vi "CrawlingPrechargeState.vi"(8 "error in (no error)":errorcluster, 9 "Cluster in":T2, 10 "Enum in":T1, 11 "Actual Start [i]":i64) -> (0 "error out":errorcluster, 2 "Cluster out":T2, 3 "Enum":T1)   [LabVIEW 2018]
uses:
  Type_Def/Type_Def Actuator Controls.ctl
  Type_Def/Type_Def ControlState.ctl
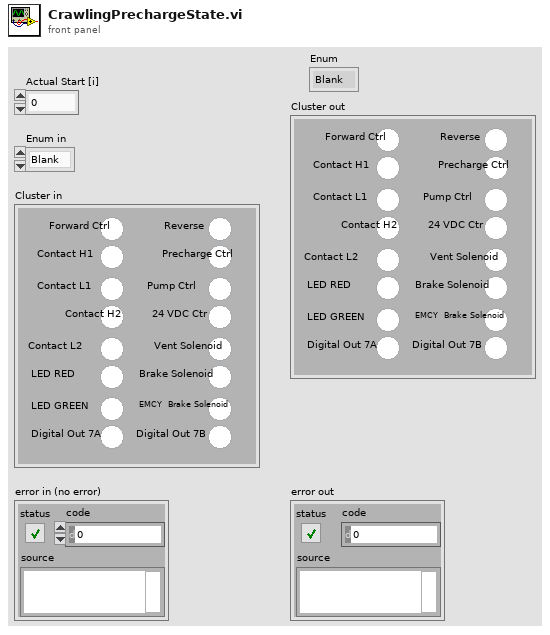
[diagram p1: front panel]
types:
  T1 = typedef "Type_Def ControlState.ctl" = enum16{"Blank", "Systems Check", "Idle", "Ready", "Pushing", "CrawlingPrecharge", "Braking", "Fault", "Boot Up", "Unpowered", "Crawling", "Shutdown", "Service Push", "Service Wait", "Vent", "Precharge"}
  T2 = typedef "Type_Def Actuator Controls.ctl" = cluster{"Reverse ":bool, "Precharge Ctrl":bool, "Pump Ctrl":bool, "24 VDC Ctr":bool, "Vent Solenoid":bool, "Brake Solenoid":bool, "EMCY  Brake Solenoid":bool, "Digital Out 7B ":bool, "Forward Ctrl":bool, "Contact H1":bool, "Contact L1":bool, "Contact H2":bool, "Contact L2 ":bool, "LED RED":bool, "LED GREEN":bool, " Digital Out 7A":bool}
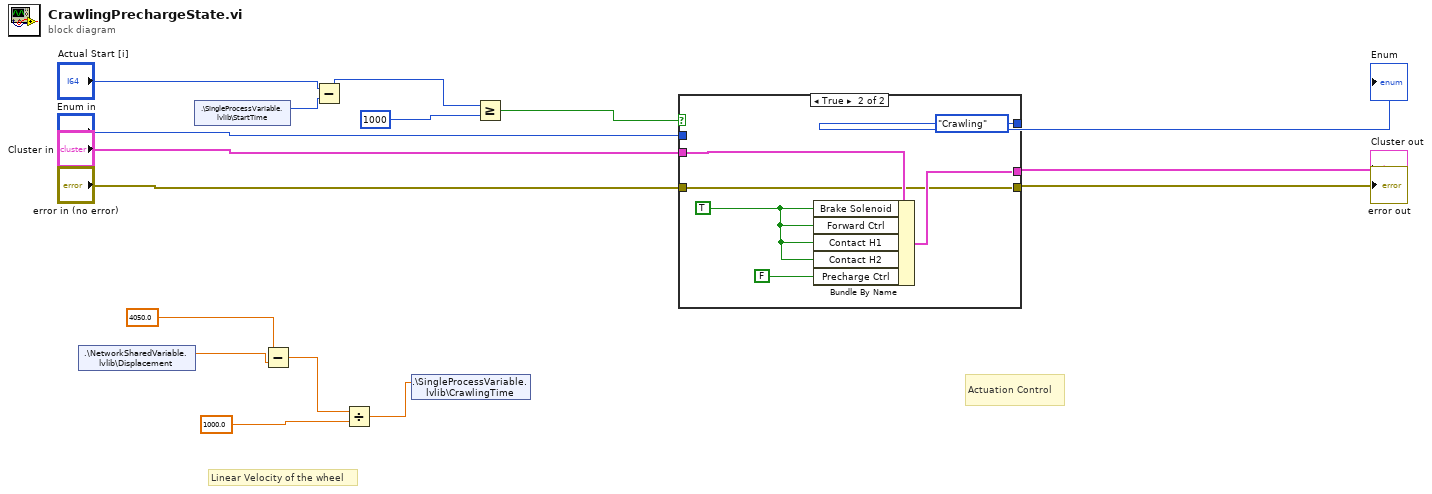
[diagram p0: block diagram]
diagram:
  # "Linear Velocity of the wheel"
  # "Actuation Control"
  n1 = shared-variable ".\\NetworkSharedVariable.lvlib\\Displacement"() -> (w14:dbl)  [unwired: 1 in, 1 out]
  n2 = shared-variable ".\\SingleProcessVariable.lvlib\\StartTime"() -> (w8:i64)  [unwired: 1 in, 1 out]
  n3 = Subtract(x=4050.0, y=w14) -> (x-y=w15:dbl)
  n4 = Subtract(x="Actual Start [i]", y=w8) -> (x-y=w10:i64)
  n5 = Divide(x=w15, y=1000.0) -> (x/y=w1:dbl)
  n6 = shared-variable ".\\SingleProcessVariable.lvlib\\CrawlingTime"(w1) -> ()  [unwired: 1 in, 1 out]
  n7 = Greater Or Equal?(x=w10, y=i64 1000) -> (x >= y?=w12:bool)
  n8 = case shown="True" w12 {
    tunnel: "Enum in" -> [w19 _]
    tunnel: [w19 Type_Def_ControlState."Crawling"] -> w3
    tunnel: "Cluster in" -> [w18 w24]
    tunnel: [w18 w23] -> w5
    tunnel: [w17 w22] -> w6
    tunnel: "error in (no error)" -> [w17 w22]
    frame False {
    }
    frame True {
      w20 = TRUE ("Digital Out 5")
      n9 = Bundle By Name(cluster=w24, "Brake Solenoid"=w20, "Forward Ctrl"=w20, "Contact H1"=w20, "Contact H2"=w20, "Precharge Ctrl"=FALSE ("Digital Out 5")) -> (w23:T2)
    }
  }
  "error out" <- w6
  "Cluster out" <- w5
  "Enum" <- w3
